vi "Serial_Analyzer_Main.vi"() -> ()   [LabVIEW 2011]
uses:
  Host/Utilities/Program Control/RS485 Settings Top Level.ctl
  Host/Utilities/FP Updates/Controls/FP Ref Enum.ctl
  Host/Utilities/FP Updates/Controls/FP Ref Cluster.ctl
  Host/Driver/Serial RS485/Controls/Serial_Action_Enum.ctl
  Host/Utilities/Data Manager/Controls/Data Manager Action.ctl
  <vilib>/Platform/TimedLoop/XDataNode/timing_clust.ctl
  <vilib>/Platform/TimedLoop/XDataNode/nitl_modes.ctl
  <vilib>/Platform/TimedLoop/XDataNode/wakeup.ctl
  Host/Utilities/System Status/System Status Enum.ctl
  <vilib>/Platform/TimedLoop/XDataNode/XDataNode.xnode
  <vilib>/Platform/TimedLoop/XDataNode/XDNodeRunTimeDep.lvlib
panel:
  out "Error OUT":errorcluster={"status"=TRUE, "code"=-63195, "source"="Read/Write Control in _RS485 Driver.vi->Serial_Analyzer_Main.vi"}
  in  "Error IN":errorcluster
  in  "Stop":bool
  in  "Start":bool
  out "RIO Comm OK":bool=TRUE
  in  "Log":bool
  in  "Clear":bool
  in  "Pause Button":bool
  in  "RS485 Settings":T1=[{"Clock Source"=FALSE, "Clock Speed (Hz)"=9600}, {"Clock Source"=FALSE, "Clock Speed (Hz)"=9600}, {"Clock Source"=FALSE, "Clock Speed (Hz)"=9600}, {"Clock Source"=FALSE, "Clock Speed (Hz)"=9600}]
  out "Results Table":string[][](table)=[["14:37:05.122", "14:37:05.008", "3", "2", "AABB", "CCEE", "", "", "", ""], ["14:37:05.122", "14:37:05.008", "4", "5", "0000", "0000", "0000", "0000", "0000", "0"], ["14:37:09.122", "14:37:09.009", "3", "2", "AABB", "CCEE", "", "", "", ""], ["14:37:09.122", "14:37:09.009", "4", "5", "0000", "0000", "0000", "0000", "0000", "0"], ["14:37:13.121", "14:37:13.009", "3", "2", "AABB", "CCEE", "", "", "", ""], ["14:37:13.121", "14:37:13.009", "4", "5", "0000", "0000", "0000", "0000", "0000", "0"], ["14:37:17.122", "14:37:17.009", "3", "2", "AABB", "CCEE", "", "", "", ""], ["14:37:17.122", "14:37:17.009", "4", "5", "0000", "0000", "0000", "0000", "0000", "0"], ["14:37:21.121", "14:37:21.009", "3", "2", "AABB", "CCEE", "", "", "", ""], ["14:37:21.121", "14:37:21.009", "4", "5", "0000", "0000", "0000", "0000", "0000", "0"], ["14:37:25.122", "14:37:25.009", "3", "2", "AABB", "CCEE", "", "", "", ""], ["14:37:25.122", "14:37:25.009", "4", "5", "0000", "0000", "0000", "0000", "0000", "0"], ["14:37:29.122", "14:37:29.010", "3", "2", "AABB", "CCEE", "", "", "", ""], ["14:37:29.122", "14:37:29.010", "4", "5", "0000", "0000", "0000", "0000", "0000", "0"], ["14:37:33.122", "14:37:33.009", "3", "2", "AABB", "CCEE", "", "", "", ""], ["14:37:33.122", "14:37:33.009", "4", "5", "0000", "0000", "0000", "0000", "0000", "0"], ["14:37:37.122", "14:37:37.010", "3", "2", "AABB", "CCEE", "", "", "", ""], ["14:37:37.122", "14:37:37.010", "4", "5", "0000", "0000", "0000", "0000", "0000", "0"], ["14:37:41.122", "14:37:41.010", "3", "2", "AABB", "CCEE", "", "", "", ""], ["14:37:41.122", "14:37:41.010", "4", "5", "0000", "0000", "0000", "0000", "0000", "0"], ["14:37:45.122", "14:37:45.010", "3", "2", "AABB", "CCEE", "", "", "", ""], ["14:37:45.122", "14:37:45.010", "4", "5", "0000", "0000", "0000", "0000", "0000", "0"], ["14:37:49.123", "14:37:49.011", "3", "2", "AABB", "CCEE", "", "", "", ""], ["14:37:49.123", "14:37:49.011", "4", "5", "0000", "0000", "0000", "0000", "0000", "0"], ["14:37:53.122", "14:37:53.010", "3", "2", "AABB", "CCEE", "", "", "", ""], ["14:37:53.122", "14:37:53.010", "4", "5", "0000", "0000", "0000", "0000", "0000", "0"], ["14:37:57.123", "14:37:57.011", "3", "2", "AABB", "CCEE", "", "", "", ""], ["14:37:57.123", "14:37:57.011", "4", "5", "0000", "0000", "0000", "0000", "0000", "0"], ["14:38:01.123", "14:38:01.011", "3", "2", "AABB", "CCEE", "", "", "", ""], ["14:38:01.123", "14:38:01.011", "4", "5", "0000", "0000", "0000", "0000", "0000", "0"], ["14:38:05.123", "14:38:05.011", "3", "2", "AABB", "CCEE", "", "", "", ""], ["14:38:05.123", "14:38:05.011", "4", "5", "0000", "0000", "0000", "0000", "0000", "0"], ["14:38:09.124", "14:38:09.011", "3", "2", "AABB", "CCEE", "", "", "", ""], ["14:38:09.124", "14:38:09.011", "4", "5", "0000", "0000", "0000", "0000", "0000", "0"], ["14:38:13.123", "14:38:13.011", "3", "2", "AABB", "CCEE", "", "", "", ""], ["14:38:13.123", "14:38:13.011", "4", "5", "0000", "0000", "0000", "0000", "0000", "0"]]
  in  "Exit":bool
  # "High Speed Serial Analyzer"
  # "Rail 1"
  # "Rail 2"
  # "Rail 3"
  # "Rail 4"
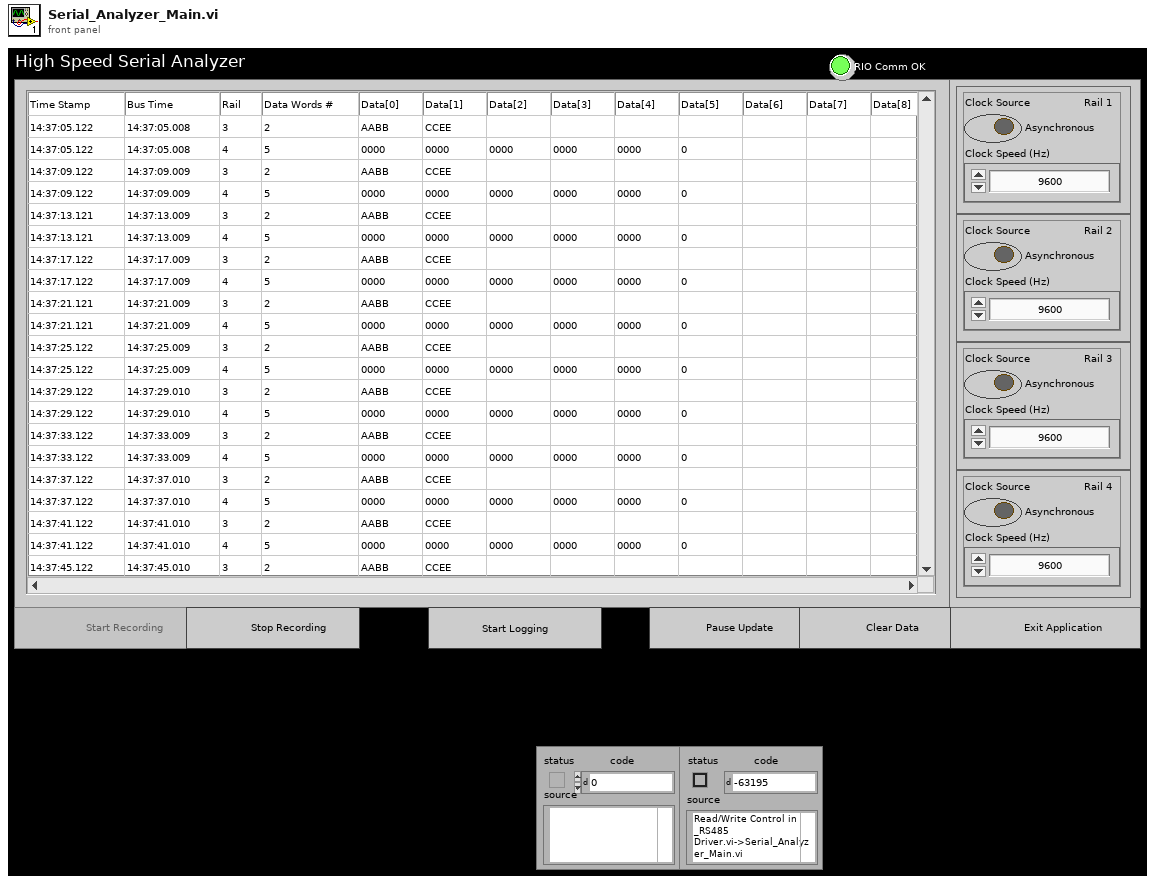
[diagram p1: front panel]
types:
  T1 = typedef "RS485 Settings Top Level.ctl" = cluster{"Clock Source":bool, "Clock Speed (Hz)":u32}[]
  T2 = typedef "FP Ref Enum.ctl" = enum16{"Get References", "Status", "Init", "Start Recording", "Stop Recording", "Pause Update", "Resume Update"}
  T3 = typedef "FP Ref Cluster.ctl" = cluster{"Start":refnum<vi>, "Stop":refnum<vi>, "Pause ":refnum<vi>, "Clear":refnum<vi>, "Exit":refnum<vi>, "Settings":refnum<vi>, "Log":refnum<vi>}
  T4 = typedef "Serial_Action_Enum.ctl" = enum16{"Init", "Status", "Close", "Read All Chan", "Set Read Start Bit", "Clear Read Start Bit", "Read Beat", "Set RS485 Settings", "Close Ref"}
  T5 = typedef "Data Manager Action.ctl" = enum16{"Init", "Status", "Get Data", "Get Log File Path", "Write Header", "Log Data", "Clear Table Data"}
  T6 = typedef "XDNodeRunTimeDep.lvlib/timing_clust.ctl" = cluster{"Expected End [f-1]":u64, "Actual End [f-1]":u64, "Finished Late? [f-1]":bool, "Expected End [i-1]":u64, "Actual End [i-1]":u64, "Finished Late? [i-1]":bool, "Expected Start [i]":u64, "Actual Start [i]":u64, "Expected Start [f]":u64, "Actual Start [f]":u64, "Source Name":string, "Structure Name":string, "Period":i64, "Deadline":i64, "Offset":i64, "Start":i64, "Priority":i32, "Timeout":i32, "Mode":T7, "Wakeup Reason":T8, "Error":errorcluster, "Source Type":string, "Secondary Source Type":string, "Global End Time":u64, "Global Start Time":u64, "Frame Duration":u64, "Iteration Duration":u64, "Assigned CPU":i32, "I/O Scan Engine Mode":u32}
  T7 = typedef "XDNodeRunTimeDep.lvlib/nitl_modes.ctl" = enum32{"No Change", "Process missed periods, maintain original phase", "Discard missed periods, maintain original phase", "Process missed periods, ignore original phase", "Discard missed periods, ignore original phase"}
  T8 = typedef "XDNodeRunTimeDep.lvlib/wakeup.ctl" = enum32{"Normal", "Aborted", "Asynchronous wakeup", "Timing source error", "Timed loop error", "Timeout"}
  T9 = typedef "System Status Enum.ctl" = enum16{"Start Recording", "Stop Recording", "Log", "Stop Log", "Pause Update", "Resume Update", "Status", "Init"}
  T10 = typedef "System Status Boolean.ctl" = cluster{"Start Recording":bool, "Log":bool, "Pause Update":bool}
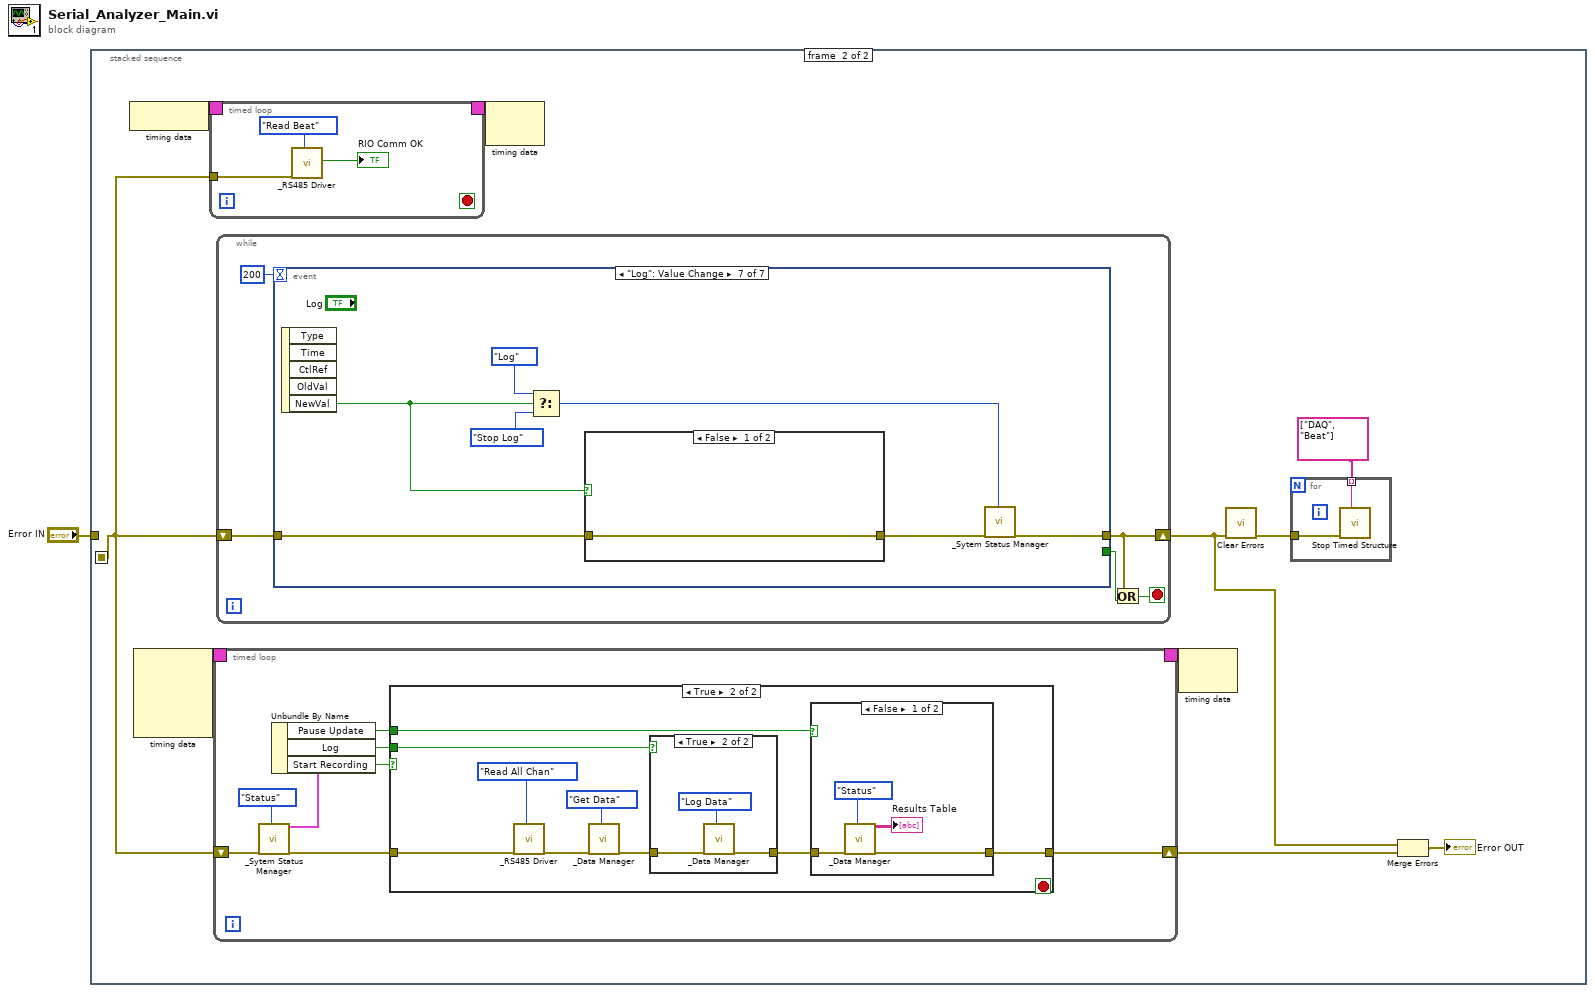
[diagram p0: block diagram]
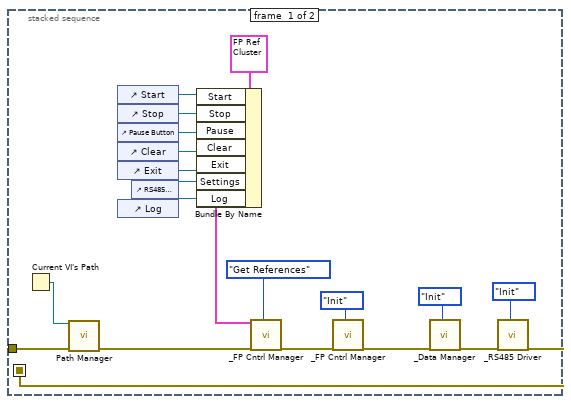
[diagram p2: hidden frame]
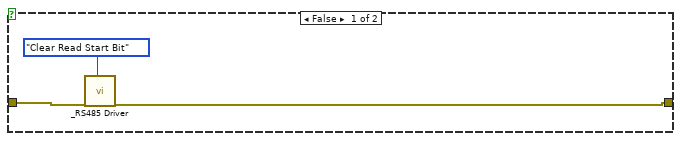
[diagram p3: hidden frame]
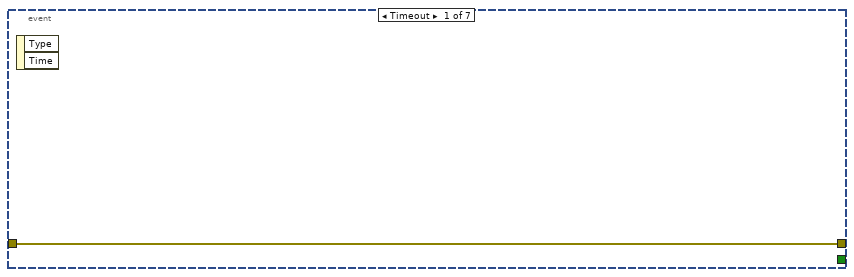
[diagram p6: hidden frame]
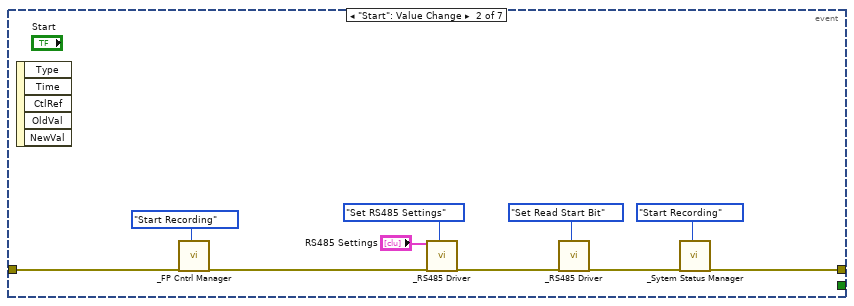
[diagram p7: hidden frame]
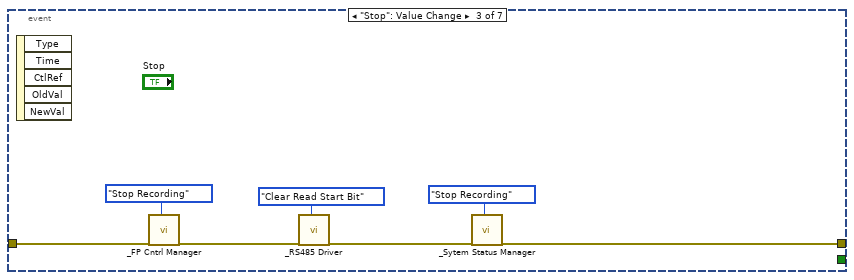
[diagram p8: hidden frame]
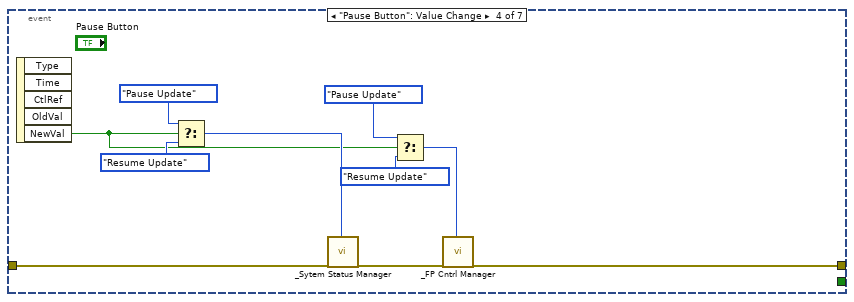
[diagram p9: hidden frame]
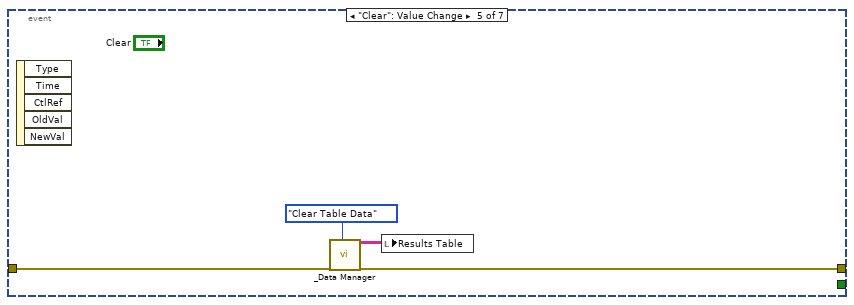
[diagram p10: hidden frame]
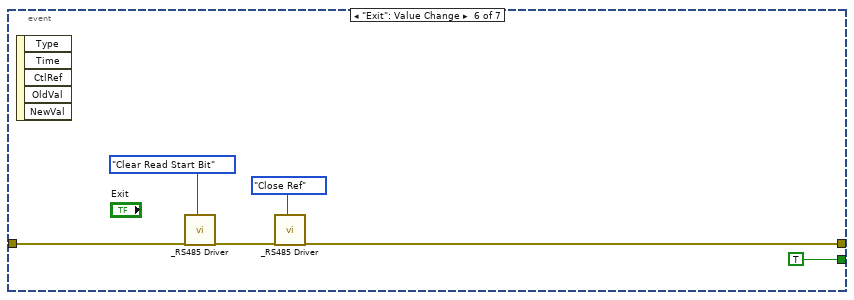
[diagram p11: hidden frame]
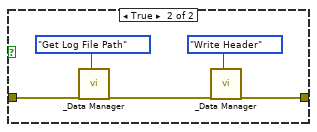
[diagram p12: hidden frame]
diagram:
  n1 = stacked-sequence {
    seq-local: [w16 _] -> [_ w22]
    tunnel: "Error IN" -> [w19 _]
    frame #0 {
      n2 = Current VI's Path() -> (path=w20:path)
      n3 = call "Path Manager.vi"("Main File Path"=w20, "Error IN"=w19) -> ("Error OUT"=w15:errorcluster)  [unwired: 12 in, 1 out]
      n4 = control-ref of="Start"() -> (w12:refnum<vi>)
      n5 = control-ref of="Stop"() -> (w11:refnum<vi>)
      n6 = control-ref of="Pause Button"() -> (w10:refnum<vi>)
      n7 = control-ref of="Clear"() -> (w9:refnum<vi>)
      n8 = control-ref of="Exit"() -> (w8:refnum<vi>)
      n9 = control-ref of="Log"() -> (w6:refnum<vi>)
      n10 = control-ref of="RS485 Settings"() -> (w7:refnum<vi>)
      n11 = Bundle By Name(cluster=T3 {"Start"=refnum, "Stop"=refnum, "Pause "=refnum, "Clear"=refnum, "Exit"=refnum, "Settings"=refnum, "Log"=refnum} ("Cluster"), "Start"=w12, "Stop"=w11, "Pause"=w10, "Clear"=w9, "Exit"=w8, "Settings"=w7, "Log"=w6) -> (w5:T3)
      n12 = call "_FP Cntrl Manager.vi"("Cluster"=w5, "Error IN"=w15, "Action"=FP_Ref_Enum."Get References") -> ("Error OUT"=w4:errorcluster)  [unwired: 16 in]
      n13 = call "_FP Cntrl Manager.vi"("Error IN"=w4, "Action"=FP_Ref_Enum."Init") -> ("Error OUT"=w3:errorcluster)  [unwired: 17 in]
      n14 = call "_Data Manager.vi"("Error IN"=w3, "Action"=Data_Manager_Action."Init") -> ("Error OUT"=w17:errorcluster)  [unwired: 16 in, 1 out]
      n15 = call "_RS485 Driver.vi"("Error IN"=w17, "Action"=Serial_Action_Enum."Init") -> ("Error OUT"=w16:errorcluster)  [unwired: 15 in, 2 out]
    }
    frame #1 {
      n16 = node-c288() -> (w29:T6)
      n17 = node-c288() -> (w31:T6)  [unwired: 4 in]
      n18 = timed-loop {
        tunnel: w22 -> [w35]
        timing: w29 -> [_]
        timing-out: [_] -> w28
        stop <- _ stop-if-true
        n19 = call "_RS485 Driver.vi"("Error IN"=w35, "Action"=Serial_Action_Enum."Read Beat") -> ("Beat"=→"RIO Comm OK":bool)  [unwired: 15 in, 2 out]
      }
      n20 = timed-loop {
        shift-right: [w43] -> w27
        shift-left: w22 -> [w47]
        timing: w31 -> [_]
        timing-out: [_] -> w30
        stop <- _ stop-if-true
        n21 = call "_Sytem Status Manager.vi"("Error IN"=w47, "Action"=System_Status_Enum."Status") -> ("Status"=w45:T10, "Error OUT"=w48:errorcluster)  [unwired: 16 in]
        n22 = Unbundle By Name(w45) -> ("Pause Update"=w41:bool, "Log"=w42:bool, "Start Recording"=w44:bool)
        n23 = case shown="True" w44 {
          tunnel: w48 -> [w50 w52]
          tunnel: [w49 w55] -> w43
          tunnel: w42 -> [_ w56]
          tunnel: w41 -> [_ w53]
          frame False {
            n24 = call "_RS485 Driver.vi"("Error IN"=w50, "Action"=Serial_Action_Enum."Clear Read Start Bit") -> ("Error OUT"=w49:errorcluster)  [unwired: 15 in, 2 out]
          }
          frame True {
            n25 = call "_RS485 Driver.vi"("Error IN"=w52, "Action"=Serial_Action_Enum."Read All Chan") -> ("Error OUT"=w60:errorcluster)  [unwired: 15 in, 2 out]
            n26 = call "_Data Manager.vi"("Error IN"=w60, "Action"=Data_Manager_Action."Get Data") -> ("Error OUT"=w58:errorcluster)  [unwired: 16 in, 1 out]
            n27 = case shown="True" w56 {
              tunnel: w58 -> [w66 w69]
              tunnel: [w66 w67] -> w54
              frame False {
              }
              frame True {
                n28 = call "_Data Manager.vi"("Error IN"=w69, "Action"=Data_Manager_Action."Log Data") -> ("Error OUT"=w67:errorcluster)  [unwired: 16 in, 1 out]
              }
            }
            n29 = case shown="False" w53 {
              tunnel: [w63 w65] -> w55
              tunnel: w54 -> [w62 w65]
              frame False {
                n30 = call "_Data Manager.vi"("Error IN"=w62, "Action"=Data_Manager_Action."Status") -> ("Table"=→"Results Table":string[][], "Error OUT"=w63:errorcluster)  [unwired: 16 in]
              }
              frame True {
              }
            }
          }
        }
      }
      n31 = while {
        shift-right: [w75] -> w24
        shift-left: w22 -> [w78]
        stop <- w76 stop-if-true
        n32 = event shown="[6] \"Log\": Value Change" {
          selector: _ -> [_ _ _ _ _ _ _]
          dyn-events: _ -> [_ _ _ _ _ _ _]
          timeout: 200 -> [_ _ _ _ _ _ _]
          tunnel: w78 -> [w79 w82 w91 w103 w109 w112 w119]
          tunnel: [w79 w83 w95 w101 w108 w115 w123] -> w75
          tunnel: [_ _ _ _ _ TRUE _] -> w74
          event Timeout {
            n33 = event-data() -> ()  [unwired: 1 in, 2 out]
          }
          event "Start": Value Change {
            n34 = event-data() -> ()  [unwired: 1 in, 5 out]
            n35 = call "_FP Cntrl Manager.vi"("Error IN"=w82, "Action"=FP_Ref_Enum."Start Recording") -> ("Error OUT"=w81:errorcluster)  [unwired: 17 in]
            n36 = call "_RS485 Driver.vi"("RS485 Settings"="RS485 Settings", "Error IN"=w81, "Action"=Serial_Action_Enum."Set RS485 Settings") -> ("Error OUT"=w85:errorcluster)  [unwired: 14 in, 2 out]
            n37 = call "_RS485 Driver.vi"("Error IN"=w85, "Action"=Serial_Action_Enum."Set Read Start Bit") -> ("Error OUT"=w84:errorcluster)  [unwired: 15 in, 2 out]
            n38 = call "_Sytem Status Manager.vi"("Error IN"=w84, "Action"=System_Status_Enum."Start Recording") -> ("Error OUT"=w83:errorcluster)  [unwired: 16 in, 1 out]
          }
          event "Stop": Value Change {
            n39 = event-data() -> ()  [unwired: 1 in, 5 out]
            n40 = call "_FP Cntrl Manager.vi"("Error IN"=w91, "Action"=FP_Ref_Enum."Stop Recording") -> ("Error OUT"=w90:errorcluster)  [unwired: 17 in]
            n41 = call "_RS485 Driver.vi"("Error IN"=w90, "Action"=Serial_Action_Enum."Clear Read Start Bit") -> ("Error OUT"=w94:errorcluster)  [unwired: 15 in, 2 out]
            n42 = call "_Sytem Status Manager.vi"("Error IN"=w94, "Action"=System_Status_Enum."Stop Recording") -> ("Error OUT"=w95:errorcluster)  [unwired: 16 in, 1 out]
          }
          event "Pause Button": Value Change {
            n43 = event-data() -> ("NewVal"=w100:bool)  [unwired: 1 in, 4 out]
            n44 = Select(t=System_Status_Enum."Pause Update" ("Action"), s=w100, f=System_Status_Enum."Resume Update" ("Action")) -> (s? t:f=w104:T9)
            n45 = call "_Sytem Status Manager.vi"("Error IN"=w103, "Action"=w104) -> ("Error OUT"=w102:errorcluster)  [unwired: 16 in, 1 out]
            n46 = Select(t=FP_Ref_Enum."Pause Update" ("Action"), s=w100, f=FP_Ref_Enum."Resume Update" ("Action")) -> (s? t:f=w97:T2)
            n47 = call "_FP Cntrl Manager.vi"("Error IN"=w102, "Action"=w97) -> ("Error OUT"=w101:errorcluster)  [unwired: 17 in]
          }
          event "Clear": Value Change {
            n48 = event-data() -> ()  [unwired: 1 in, 5 out]
            n49 = call "_Data Manager.vi"("Error IN"=w109, "Action"=Data_Manager_Action."Clear Table Data") -> ("Table"=w107:string[][], "Error OUT"=w108:errorcluster)  [unwired: 16 in]
            n50 = local write "Results Table"(w107) -> ()
          }
          event "Exit": Value Change {
            n51 = event-data() -> ()  [unwired: 1 in, 5 out]
            n52 = call "_RS485 Driver.vi"("Error IN"=w112, "Action"=Serial_Action_Enum."Clear Read Start Bit") -> ("Error OUT"=w111:errorcluster)  [unwired: 15 in, 2 out]
            n53 = call "_RS485 Driver.vi"("Error IN"=w111, "Action"=Serial_Action_Enum."Close Ref") -> ("Error OUT"=w115:errorcluster)  [unwired: 15 in, 2 out]
          }
          event "Log": Value Change {
            n54 = event-data() -> ("NewVal"=w117:bool)  [unwired: 1 in, 4 out]
            n55 = Select(t=System_Status_Enum."Log" ("Action"), s=w117, f=System_Status_Enum."Stop Log" ("Action")) -> (s? t:f=w120:T9)
            n56 = case shown="False" w117 {
              tunnel: w119 -> [w124 w128]
              tunnel: [w124 w125] -> w118
              frame False {
              }
              frame True {
                n57 = call "_Data Manager.vi"("Error IN"=w128, "Action"=Data_Manager_Action."Get Log File Path") -> ("Error OUT"=w126:errorcluster)  [unwired: 16 in, 1 out]
                n58 = call "_Data Manager.vi"("Error IN"=w126, "Action"=Data_Manager_Action."Write Header") -> ("Error OUT"=w125:errorcluster)  [unwired: 16 in, 1 out]
              }
            }
            n59 = call "_Sytem Status Manager.vi"("Error IN"=w118, "Action"=w120) -> ("Error OUT"=w123:errorcluster)  [unwired: 16 in, 1 out]
          }
        }
        n60 = Or(x=w75, y=w74) -> (x .or. y?=w76:bool)
      }
      n61 = node-c288(w28) -> ()  [unwired: 1 out]
      n62 = node-c288(w30) -> ()  [unwired: 1 out]
      n63 = call <vilib>:"Clear Errors.vi"("error in (no error)"=w24) -> ("error out"=w25:errorcluster)  [unwired: 6 in]
      n64 = for {
        tunnel: w25 -> [w33]
        tunnel: string[] ["DAQ", "Beat"] -> [w32] mode=indexing
        n65 = call <vilib>:"Stop Timed Structure.vi"("error in (no error)"=w33, "name"=w32) -> ()  [unwired: 9 in, 1 out]
      }
      n66 = Merge Errors(w24, w27) -> (→"Error OUT":errorcluster)
    }
  }
